vi "Configure.vi"(8 "error in (no error)":errorcluster, 11 "DataLogger in":refnum<class "DataLogger.lvclass">) -> (0 "error out":errorcluster, 3 "DataLogger out":refnum<class "DataLogger.lvclass">)   [LabVIEW 2020, in "datalogger.lvlib" / "DataLogger.lvclass"]
uses:
  DataLogger.lvclass
  DataLogger.lvclass/DataLogger.ctl
  Hardware Abstraction Layer/Component/GenericActor/GenericActor/GenericActor.lvclass
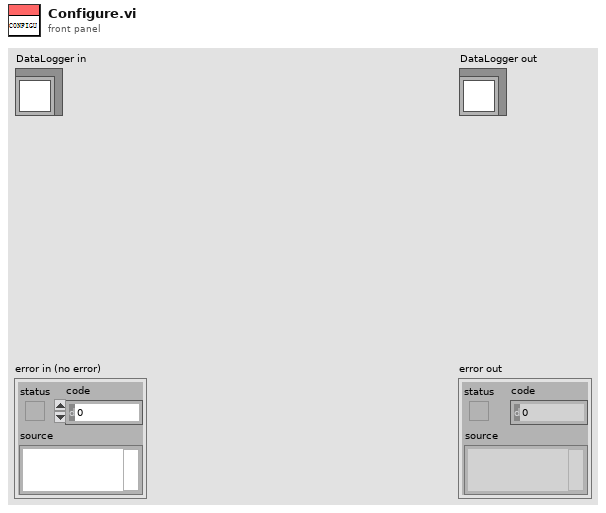
[diagram p1: front panel]
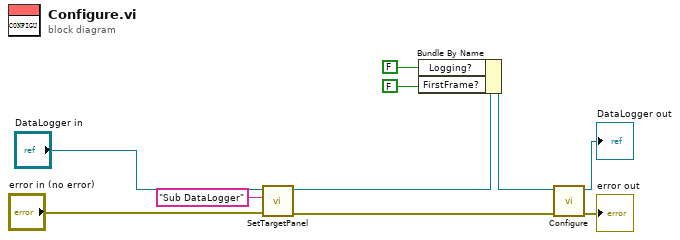
[diagram p0: block diagram]
diagram:
  n1 = call-dynamic "SetTargetPanel.vi"("error in (no error)"="error in (no error)", "TargetPanel"="Sub DataLogger" ("Panel"), "GRMActor in"="DataLogger in") -> ("error out"=w7:errorcluster, "GRMActor out"=w5:refnum<class "DataLogger.lvclass">)  [unwired: 7 in]
  n2 = Bundle By Name(cluster=w5, "Logging?"=FALSE, "FirstFrame?"=FALSE) -> (w3:refnum<class "DataLogger.lvclass">)
  n3 = call-parent "Configure.vi"("error in (no error)"=w7, "GRMActor in"=w3) -> ("error out"=→"error out":errorcluster, "GRMActor out"=→"DataLogger out":refnum<class "DataLogger.lvclass">)  [unwired: 8 in]
